vi "motor string cluster to numeric array.vi"(1 "Motor Positions Actual":T1) -> (0 "Array":dbl[](array[numeric]))   [LabVIEW 2011]
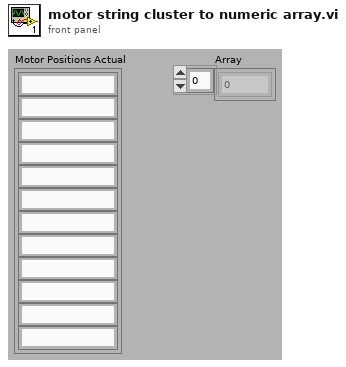
[diagram p1: front panel]
types:
  T1 = cluster{string, string, string, string, string, string, string, string, string, string, string, string}
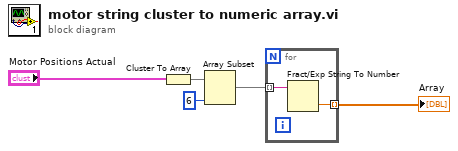
[diagram p0: block diagram]
diagram:
  n1 = Cluster To Array(cluster="Motor Positions Actual") -> (array=w2:string[])
  n2 = Array Subset(array=w2, length=6) -> (w4:string[])  [unwired: 1 in]
  n3 = for {
    tunnel: w4 -> [w7] mode=indexing
    tunnel: [w6] -> w5 mode=indexing
    n4 = Fract/Exp String To Number(string=w7) -> (number=w6:dbl)  [unwired: 3 in, 1 out]
  }
  "Array" <- w5
